vi "Open Config.vi"(10 "Config Path":path, 11 "Test Config":T1={"Test Header"={"CA Number:"="", "Part Model:"="", "Part Serial Number:"="", "Technician Name:"="", "Test Fluid:"="", "Hours Description:"="", "Notes:"="", "Data Storage Folder:"=path ""}, "Test Style"=enum."Wet Test", "Bias Resistance"=nan, "Height Offset"=nan, "Graph Parameters"={"Tol Path"=path "", "Tol Band Color"=enum."Red", "Graph Type"=enum."H vs R (1 Cycle)", "Height Min"=0, "Height Max"=0, "Height Interval"=0, "Res Max"=0, "Res Interval"=0, "Time Max"=0, "Time Interval"=0, "Graph Output File"=enum."png", "Auto Open"=FALSE}, "Test Parameters"={"Sweep Start Height"=0.0, "Sweep End Height"=0.0, "Sweep Time (s)"=0.0, "Sweep PS Cmd"=0.0, "Number of Sweeps"=0}} {"Test Parameters"."Sweep Time (s)" min=0.0 step=0.01 format="%.2g"}) -> (3 "Test Config OUT":T1={"Test Header"={"CA Number:"="", "Part Model:"="", "Part Serial Number:"="", "Technician Name:"="", "Test Fluid:"="", "Hours Description:"="", "Notes:"="", "Data Storage Folder:"=path ""}, "Test Style"=enum."Wet Test", "Bias Resistance"=nan, "Height Offset"=nan, "Graph Parameters"={"Tol Path"=path "", "Tol Band Color"=enum."Red", "Graph Type"=enum."H vs R (1 Cycle)", "Height Min"=0, "Height Max"=0, "Height Interval"=0, "Res Max"=0, "Res Interval"=0, "Time Max"=0, "Time Interval"=0, "Graph Output File"=enum."png", "Auto Open"=FALSE}, "Test Parameters"={"Sweep Start Height"=0.0, "Sweep End Height"=0.0, "Sweep Time (s)"=0.0, "Sweep PS Cmd"=0.0, "Number of Sweeps"=0}} {"Test Parameters"."Sweep Time (s)" min=0.0 step=0.01 format="%.2g"})   [LabVIEW 2019]
uses:
  TypeDef/Test Config.ctl
  TypeDef/Test Header.ctl
  TypeDef/Test Style.ctl
  TypeDef/Graph Parameters.ctl
  TypeDef/Color.ctl
  TypeDef/Graph Type.ctl
  TypeDef/Graph Output File.ctl
  TypeDef/Test Parameters.ctl
  TypeDef/Test Config v1.ctl
  TypeDef/Test Header v1.ctl
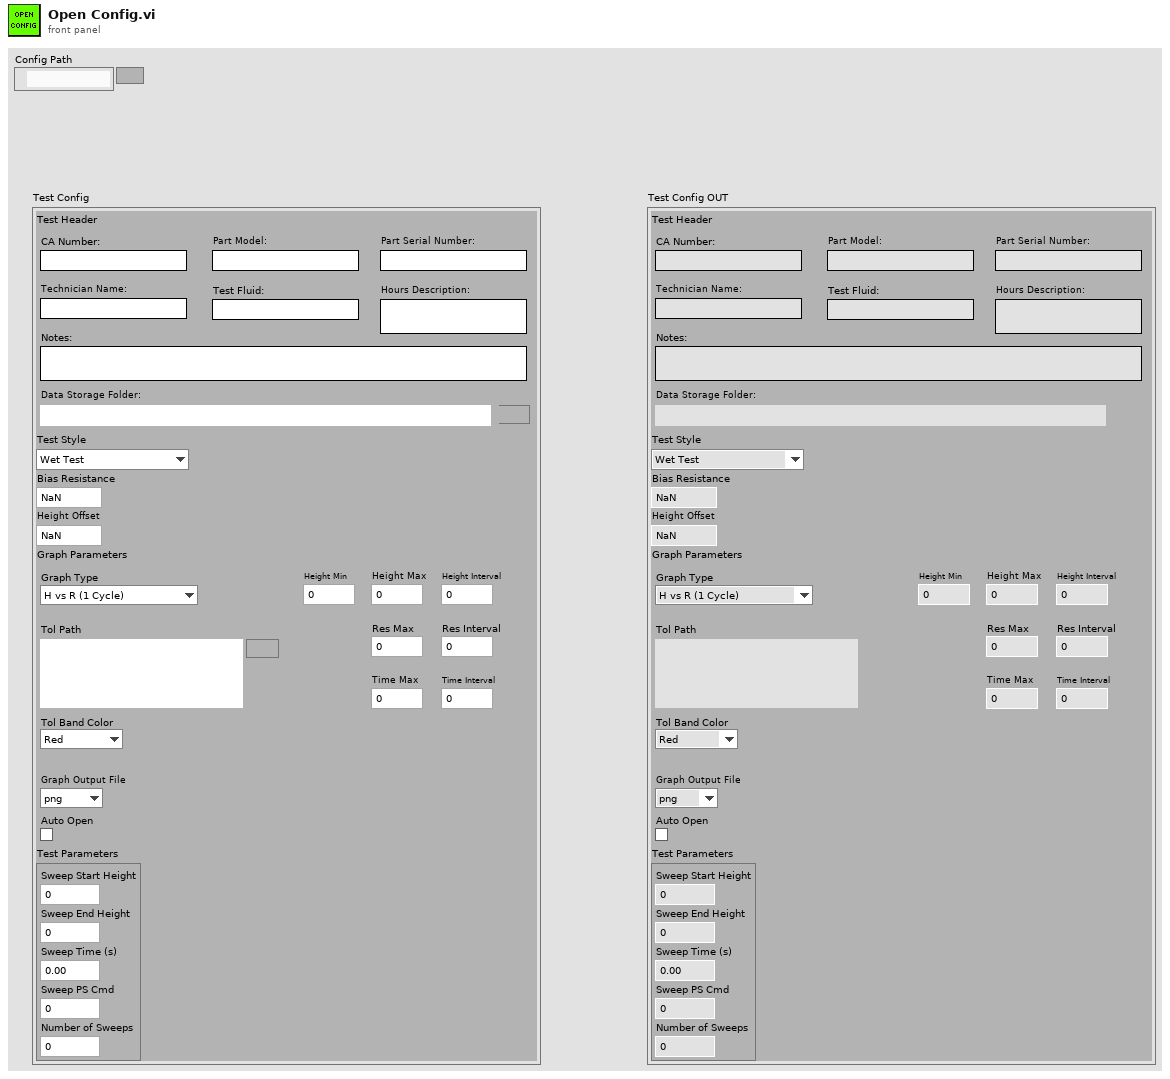
[diagram p1: front panel]
types:
  T1 = typedef "Test Config.ctl" = cluster{"Test Header":T2, "Test Style":T3, "Bias Resistance":dbl, "Height Offset":dbl, "Graph Parameters":T4, "Test Parameters":T8}
  T2 = typedef "Test Header.ctl" = cluster{"CA Number:":string, "Part Model:":string, "Part Serial Number:":string, "Technician Name:":string, "Test Fluid:":string, "Hours Description:":string, "Notes:":string, "Data Storage Folder:":path}
  T3 = typedef "Test Style.ctl" = enum16{"Wet Test", "Dry Test", "Contact Test"}
  T4 = typedef "Graph Parameters.ctl" = cluster{"Tol Path":path, "Tol Band Color":T5, "Graph Type":T6, "Height Min":i32, "Height Max":i32, "Height Interval":i32, "Res Max":i32, "Res Interval":i32, "Time Max":i32, "Time Interval":i32, "Graph Output File":T7, "Auto Open":bool}
  T5 = typedef "Color.ctl" = enum16{"Red", "Black", "Green", "Blue", "Orange", "Yellow", "Purple", "Grey"}
  T6 = typedef "Graph Type.ctl" = enum16{"H vs R (1 Cycle)", "T vs R (Multiple Cycles)", "H vs R & T vs R (1 Cycle)"}
  T7 = typedef "Graph Output File.ctl" = enum16{"png", "pdf"}
  T8 = typedef "Test Parameters.ctl" = cluster{"Sweep Start Height":dbl, "Sweep End Height":dbl, "Sweep Time (s)":dbl, "Sweep PS Cmd":dbl, "Number of Sweeps":i32}
  T9 = typedef "Test Config v1.ctl" = cluster{"Test Header":T10, "Test Style":T3, "Bias Resistance":dbl, "Height Offset":dbl, "Graph Parameters":T4, "Test Parameters":T8}
  T10 = typedef "Test Header v1.ctl" = cluster{"CA Number:":string, "Part Model:":string, "Part Serial Number:":string, "Technician Name:":string, "Test Fluid:":string, "Hours Description:":string, "Data Storage Folder:":path}
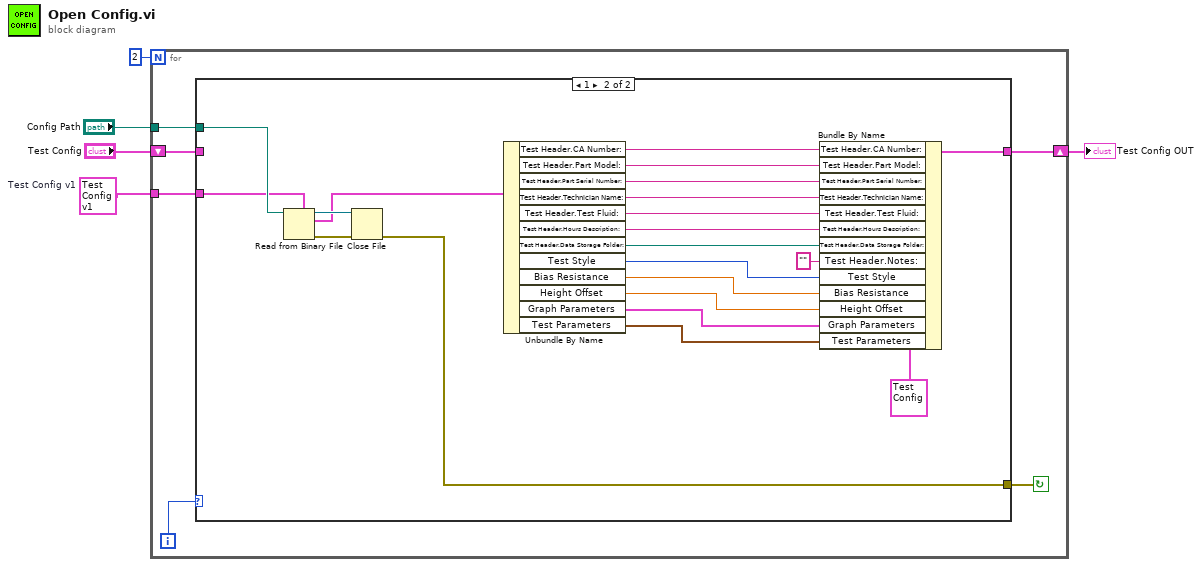
[diagram p0: block diagram]
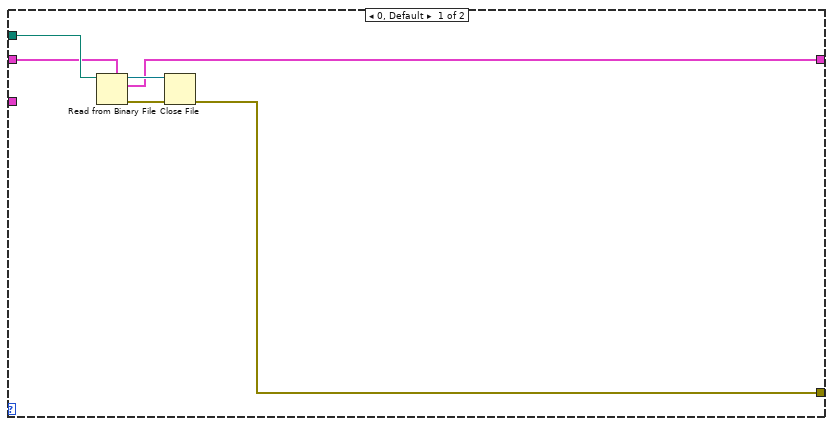
[diagram p2: hidden frame]
diagram:
  w1 = T9 {"Test Header"={"CA Number:"="", "Part Model:"="", "Part Serial Number:"="", "Technician Name:"="", "Test Fluid:"="", "Hours Description:"="", "Data Storage Folder:"=path ""}, "Test Style"=enum."Wet Test", "Bias Resistance"=nan, "Height Offset"=nan, "Graph Parameters"={"Tol Path"=path "", "Tol Band Color"=enum."Red", "Graph Type"=enum."H vs R (1 Cycle)", "Height Min"=0, "Height Max"=0, "Height Interval"=0, "Res Max"=0, "Res Interval"=0, "Time Max"=0, "Time Interval"=0, "Graph Output File"=enum."png", "Auto Open"=FALSE}, "Test Parameters"={"Sweep Start Height"=0.0, "Sweep End Height"=0.0, "Sweep Time (s)"=0.0, "Sweep PS Cmd"=0.0, "Number of Sweeps"=0}}  # Test Config v1
  n1 = for {
    N: 2 -> [_]
    tunnel: w1 -> [w9]
    tunnel: "Config Path" -> [w8]
    shift-right: [w6] -> w2
    shift-left: "Test Config" -> [w10]
    i -> [w11]
    stop <- w7 continue-if-true
    n2 = case shown="1" w11 {
      tunnel: w10 -> [w16 _]
      tunnel: w9 -> [_ w34]
      tunnel: w8 -> [w17 w38]
      tunnel: [w13 w35] -> w7
      tunnel: [w12 w33] -> w6
      frame 0, Default {
        n3 = Read from Binary File(5:w16, 11:w17) -> (0:w14:errorcluster, 2:w12:T1, 3:w15:refnum<file>)  [unwired: 4 in, 1 out]
        n4 = Close File(refnum=w15, error in=w14) -> (error out=w13:errorcluster)  [unwired: 1 out]
      }
      frame 1 {
        n5 = Read from Binary File(5:w34, 11:w38) -> (0:w36:errorcluster, 2:w32:T9, 3:w37:refnum<file>)  [unwired: 4 in, 1 out]
        n6 = Close File(refnum=w37, error in=w36) -> (error out=w35:errorcluster)  [unwired: 1 out]
        n7 = Unbundle By Name(w32) -> ("Test Header.CA Number:"=w30:string, "Test Header.Part Model:"=w29:string, "Test Header.Part Serial Number:"=w28:string, "Test Header.Technician Name:"=w27:string, "Test Header.Test Fluid:"=w26:string, "Test Header.Hours Description:"=w25:string, "Test Header.Data Storage Folder:"=w24:path, "Test Style"=w23:T3, "Bias Resistance"=w22:dbl, "Height Offset"=w21:dbl, "Graph Parameters"=w20:T4, "Test Parameters"=w19:T8)
        n8 = Bundle By Name(cluster=T1 {"Test Header"={"CA Number:"="", "Part Model:"="", "Part Serial Number:"="", "Technician Name:"="", "Test Fluid:"="", "Hours Description:"="", "Notes:"="", "Data Storage Folder:"=path ""}, "Test Style"=enum."Wet Test", "Bias Resistance"=nan, "Height Offset"=nan, "Graph Parameters"={"Tol Path"=path "", "Tol Band Color"=enum."Red", "Graph Type"=enum."H vs R (1 Cycle)", "Height Min"=0, "Height Max"=0, "Height Interval"=0, "Res Max"=0, "Res Interval"=0, "Time Max"=0, "Time Interval"=0, "Graph Output File"=enum."png", "Auto Open"=FALSE}, "Test Parameters"={"Sweep Start Height"=0.0, "Sweep End Height"=0.0, "Sweep Time (s)"=0.0, "Sweep PS Cmd"=0.0, "Number of Sweeps"=0}} ("Test Config"), "Test Header.CA Number:"=w30, "Test Header.Part Model:"=w29, "Test Header.Part Serial Number:"=w28, "Test Header.Technician Name:"=w27, "Test Header.Test Fluid:"=w26, "Test Header.Hours Description:"=w25, "Test Header.Data Storage Folder:"=w24, "Test Header.Notes:"="", "Test Style"=w23, "Bias Resistance"=w22, "Height Offset"=w21, "Graph Parameters"=w20, "Test Parameters"=w19) -> (w33:T1)
      }
    }
  }
  "Test Config OUT" <- w2
